vi "stop.vi"(8 "error in (no error)":errorcluster, 9 "CameraSettings":refnum<class "CamaraSettings.lvclass">, 10 "stop":bool, 11 "NetworkPixelfly in":refnum<class "NetworkPixelfly.lvclass">) -> (0 "error out":errorcluster, 1 "imageSaved":bool, 2 "stopped?":bool, 3 "NetworkPixelfly out":refnum<class "NetworkPixelfly.lvclass">)   [LabVIEW 2011, in "Hardware.lvlib" / "HWControllers.lvlib" / "NetworkPixelfly.lvclass"]
uses:
  NetworkPixelfly.lvclass
  Tools/CameraSettings/CamaraSettings.lvclass
  Channels/Camera/PixelflySA/PixelflySA.lvclass
  NetworkCamera.lvclass
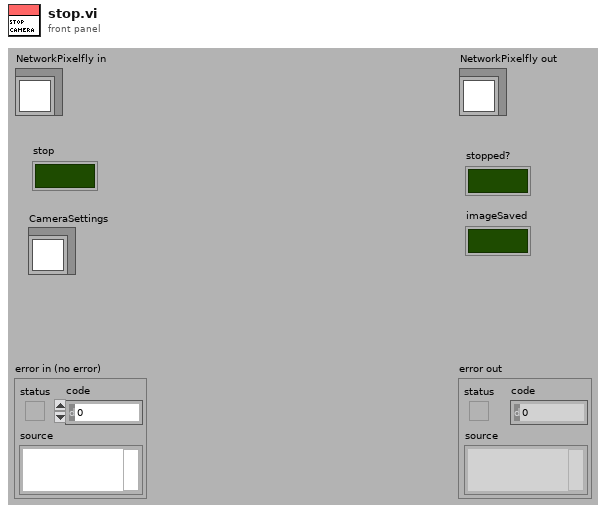
[diagram p1: front panel]
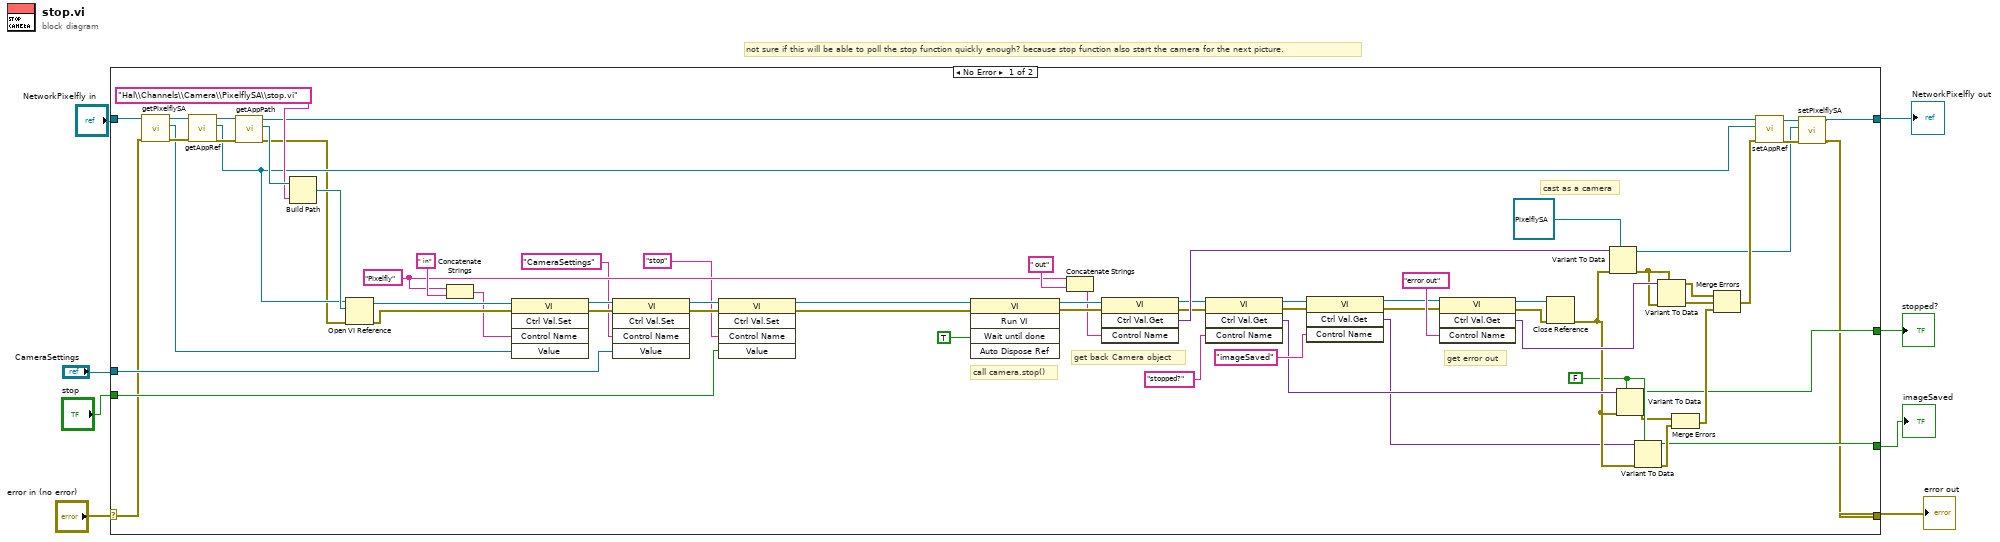
[diagram p0: block diagram]
diagram:
  # "not sure if this will be able to poll the stop function quickly enough? because stop function also start the camera for the next picture."
  n1 = case shown="No Error" "error in (no error)" {
    selector: "error in (no error)" -> [w15 w75]
    tunnel: [w11 w75] -> w7
    tunnel: [w13 w74] -> w1
    tunnel: "NetworkPixelfly in" -> [w16 w74]
    tunnel: "CameraSettings" -> [w50 _]
    tunnel: "stop" -> [w48 _]
    tunnel: [w23 _] -> w3
    tunnel: [w22 _] -> w2
    frame No Error {
      w27 = FALSE
      w58 = "Pixelfly" ("Control name")
      # "get error out"
      # "get back Camera object"
      # "call camera.stop()"
      # "cast as a camera"
      n2 = call "getPixelflySA.vi"("error in (no error)"=w15, "NetworkCamera in"=w16) -> ("error out"=w18:errorcluster, "PixelflySA.lvclass"=w17:refnum<class "PixelflySA.lvclass">, "NetworkCamera out"=w19:refnum<class "NetworkPixelfly.lvclass">)  [unwired: 7 in]
      n3 = call "getAppRef.vi"("error in (no error)"=w18, "NetworkCamera in"=w19) -> ("error out"=w61:errorcluster, "appRef"=w56:refnum<vi>, "NetworkCamera out"=w62:refnum<class "NetworkPixelfly.lvclass">)  [unwired: 7 in]
      n4 = call "getAppPath.vi"("error in (no error)"=w61, "NetworkCamera in"=w62) -> ("error out"=w39:errorcluster, "appPath"=w60:path, "NetworkCamera out"=w57:refnum<class "NetworkPixelfly.lvclass">)  [unwired: 7 in]
      n5 = Build Path(base path=w60, name or relative path="Hal\\Channels\\Camera\\PixelflySA\\stop.vi" ("viPath")) -> (appended path=w73:path)
      n6 = Open VI Reference(application reference (local)=w56, vi path=w73, error in (no error)=w39) -> (vi reference=w68:refnum<vi>, error out=w67:errorcluster)  [unwired: 3 in]
      n7 = Concatenate Strings(w58, " in") -> (w65:string)
      n8 = invoke class="VI" method="Ctrl Val.Set"(reference=w68, error in=w67, "Control Name"=w65, "Value"=w17) -> (reference out=w55:refnum<vi>, error out=w53:errorcluster)  [unwired: 1 in, 3 out]
      n9 = invoke class="VI" method="Ctrl Val.Set"(reference=w55, error in=w53, "Control Name"="CameraSettings", "Value"=w50) -> (reference out=w54:refnum<vi>, error out=w52:errorcluster)  [unwired: 1 in, 3 out]
      n10 = invoke class="VI" method="Ctrl Val.Set"(reference=w54, error in=w52, "Control Name"="stop", "Value"=w48) -> (reference out=w21:refnum<vi>, error out=w20:errorcluster)  [unwired: 1 in, 3 out]
      n11 = invoke class="VI" method="Run VI"(reference=w21, error in=w20, "Wait until done"=TRUE) -> (reference out=w71:refnum<vi>, error out=w70:errorcluster)  [unwired: 2 in, 3 out]
      n12 = Concatenate Strings(w58, " out") -> (w63:string)
      n13 = invoke class="VI" method="Ctrl Val.Get"(reference=w71, error in=w70, "Control Name"=w63) -> (reference out=w38:refnum<vi>, error out=w35:errorcluster, "Get Control Value Variant"=w69:variant)  [unwired: 1 in, 1 out]
      n14 = invoke class="VI" method="Ctrl Val.Get"(reference=w38, error in=w35, "Control Name"="stopped?") -> (reference out=w37:refnum<vi>, error out=w36:errorcluster, "Get Control Value Variant"=w30:variant)  [unwired: 1 in, 1 out]
      n15 = invoke class="VI" method="Ctrl Val.Get"(reference=w37, error in=w36, "Control Name"="imageSaved") -> (reference out=w34:refnum<vi>, error out=w33:errorcluster, "Get Control Value Variant"=w28:variant)  [unwired: 1 in, 1 out]
      n16 = invoke class="VI" method="Ctrl Val.Get"(reference=w34, error in=w33, "Control Name"="error out") -> (reference out=w47:refnum<vi>, error out=w45:errorcluster, "Get Control Value Variant"=w44:variant)  [unwired: 1 in, 1 out]
      n17 = Close Reference(reference=w47, error in (no error)=w45) -> (error out=w29:errorcluster)
      n18 = Variant To Data(error in=w29, type=refnum<class "PixelflySA.lvclass"> refnum ("PixelflySA.lvclass"), Variant=w69) -> (data=w9:refnum<class "PixelflySA.lvclass">, error out=w43:errorcluster)
      n19 = Variant To Data(error in=w29, type=w27, Variant=w30) -> (data=w23:bool, error out=w26:errorcluster)
      n20 = Variant To Data(error in=w29, type=w27, Variant=w28) -> (data=w22:bool, error out=w25:errorcluster)
      n21 = Variant To Data(error in=w43, type=w43, Variant=w44) -> (data=w42:errorcluster, error out=w41:errorcluster)
      n22 = Merge Errors(w26, w25) -> (w24:errorcluster)
      n23 = Merge Errors(w42, w41, w24) -> (w40:errorcluster)
      n24 = call "setAppRef.vi"("error in (no error)"=w40, "appRef"=w56, "NetworkCamera in"=w57) -> ("error out"=w12:errorcluster, "NetworkCamera out"=w14:refnum<class "NetworkPixelfly.lvclass">)  [unwired: 7 in]
      n25 = call "setPixelflySA.vi"("error in (no error)"=w12, "PixelflySA.lvclass"=w9, "NetworkCamera in"=w14) -> ("error out"=w11:errorcluster, "NetworkCamera out"=w13:refnum<class "NetworkPixelfly.lvclass">)  [unwired: 7 in]
    }
    frame Error {
    }
  }
  "error out" <- w7
  "NetworkPixelfly out" <- w1
  "stopped?" <- w3
  "imageSaved" <- w2
